vi "testV7-Timer.vi"() -> ()   [LabVIEW 2020]
uses:
  <vilib>/DAQmx/read.llb/DAQmx Read (Analog 2D DBL NChan NSamp).vi
  <vilib>/Analysis/baseanly.llb/Mean (DBL).vi
  <vilib>/DAQmx/miscellaneous.llb/DAQmx Fill In Error Info.vi
  <vilib>/Analysis/NI_AALBase.lvlib
  <resource>/objmgr/daqmx.rc
panel:
  out "index of element":i32
  out "element":dbl
  out "?":timestamp
  out "Channels":refnum<k21>[](array[refnum])
  in  "stop":bool
  out "size(s)":i32
  out "NumDevices":u32
  out "x/y":dbl
  in  "?":T1(tab)
  in  "Sampling Time":u32=5
  in  "Read Time (s)":u32=60
  in  "Channel List":string(combo)="Temperature"
  out "Read Count Daily":string="7/26/2020\n 6:17:48 PM" caption="Timestamp"
  out "Countdown to Read":string="7/26/2020\n 6:17:48 PM" caption="Timestamp"
  out "?":string
  out "?":string
  out "Timestamp":string="7/26/2020\n 6:17:48 PM"
  in  "Play Button 2":bool
  in  "Next Button":bool
  in  "Stop Button 2":bool
  out "Graph Running":bool
  in  "Resolution":u8=10 min=10
  in  "Stop Button":bool
  in  "Play Button":bool
  out "Module 3":bool
  out "Module 2":bool
  out "Module 1":bool
  out "3":bool
  out "2":bool
  out "1":bool
  in  "Running Module":u8=1 min=1 max=3
  in  "Module 3 Task":refnum<k21>="MyTemperatureTask_2"
  out "?":waveform(dbl)(graph)
  in  "Module 3 File Data Location":path=path "E:/KMUTT/Master Degree/labviewjgsee/log/Module3"
  in  "Module 2 File Data Location":path=path "E:/KMUTT/Master Degree/labviewjgsee/log/Module2"
  in  "Module 2 Task":refnum<k21>="MyTemperatureTask_1"
  in  "Module 1 File Data Location":path=path "E:/KMUTT/Master Degree/labviewjgsee/log/Module1"
  in  "Module 1 Task":refnum<k21>="MyTemperatureTask"
  in  "DAQmx Device Name":tag
  out "Table Module 1":string[][](table)
  out "Table Module 2":string[][](table)
  out "Table Module 3":string[][](table)
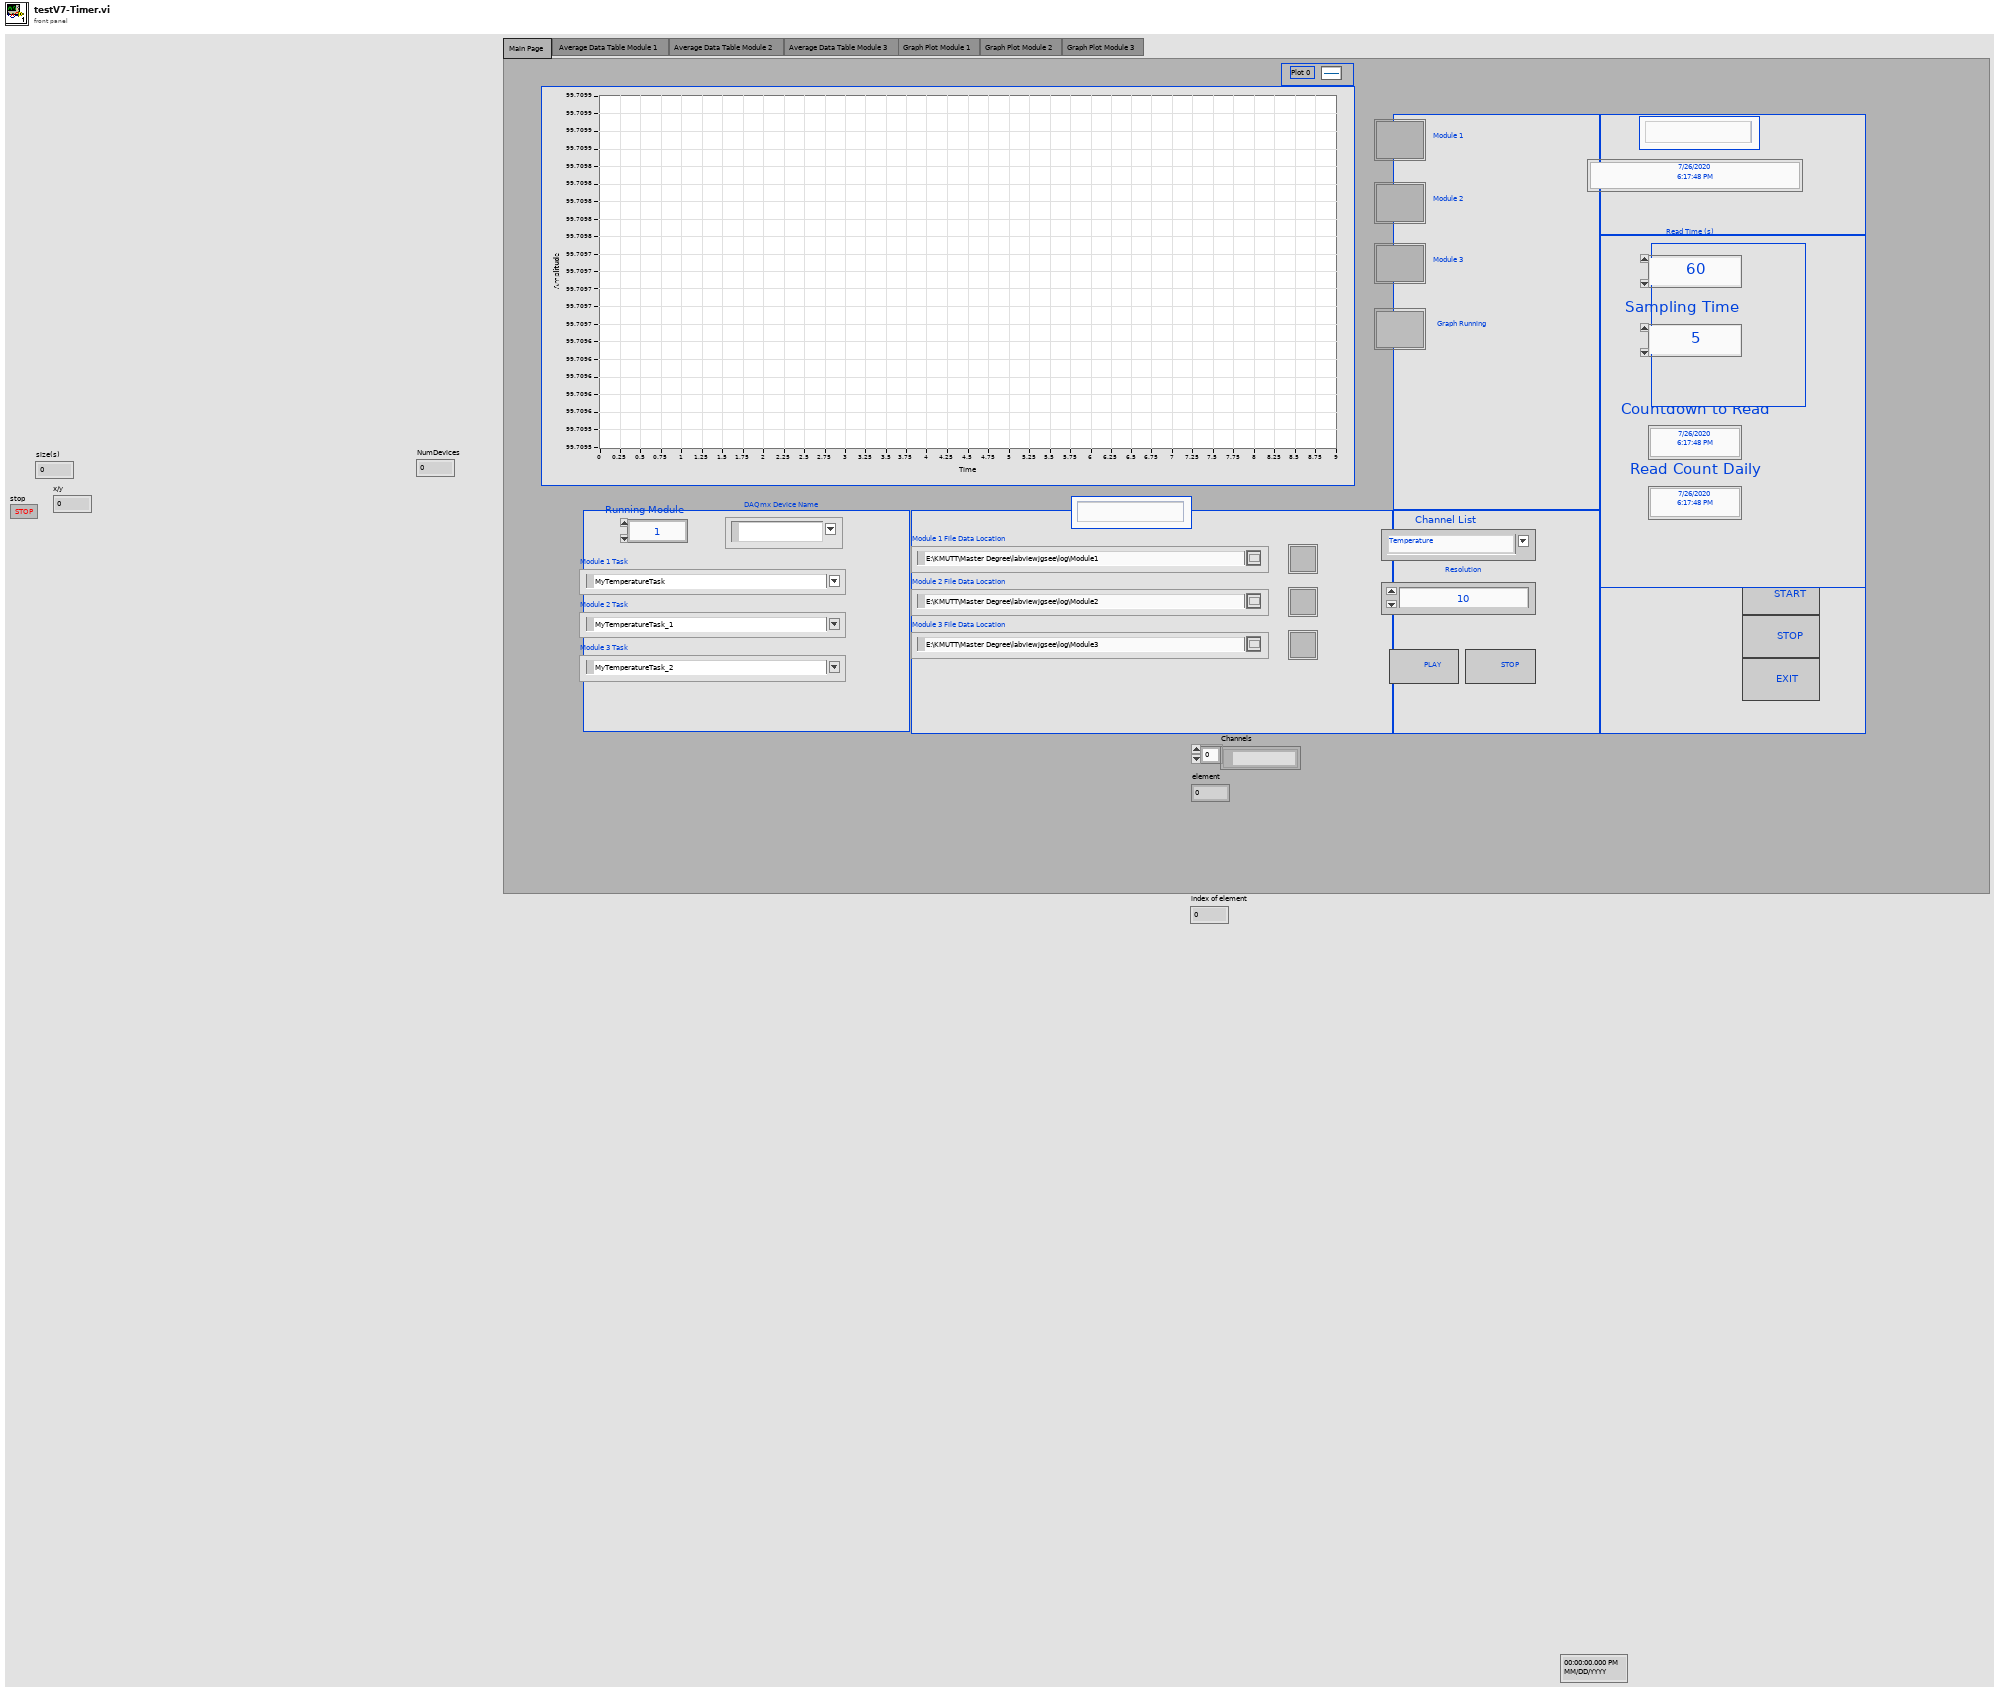
[diagram p1: front panel]
types:
  T1 = enum32{"Main Page ", " Average Data Table Module 1", "Average Data Table Module 2", "Average Data Table Module 3", "Graph Plot Module 1", "Graph Plot Module 2", "Graph Plot Module 3"}
  T2 = enum16{"open", "replace", "create", "open or create", "replace or create", "replace or create with confirmation"}
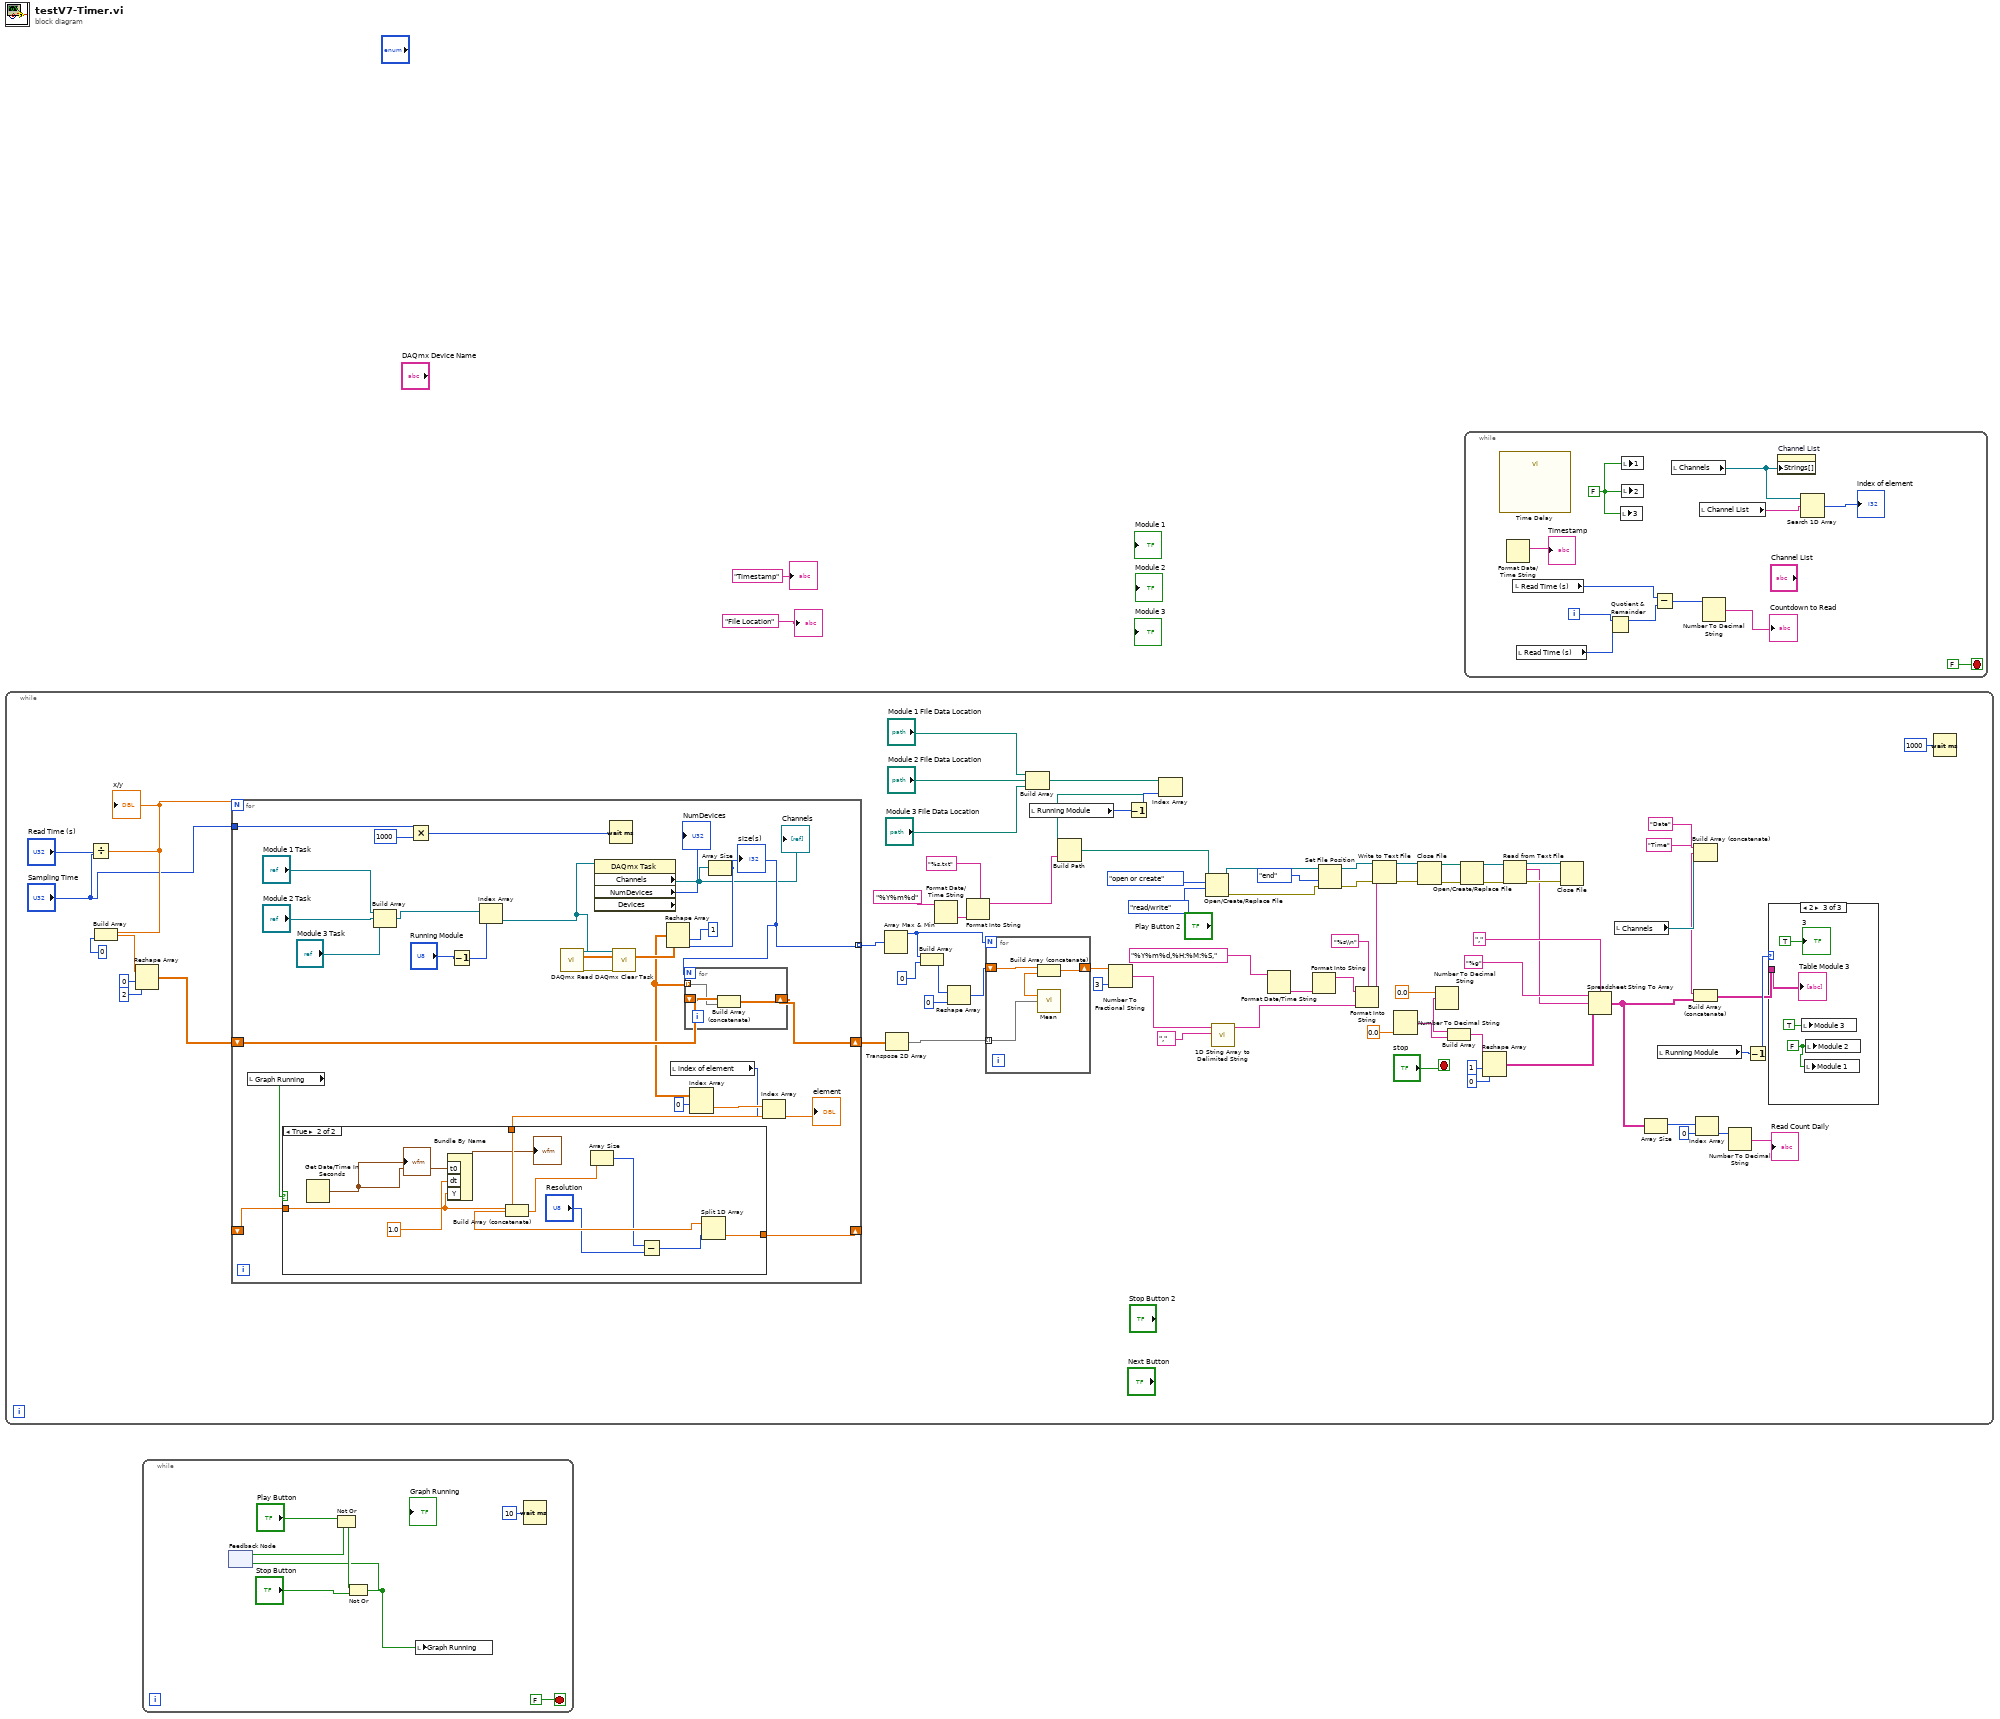
[diagram p0: block diagram]
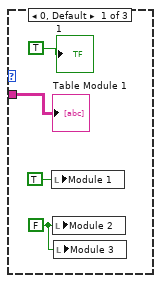
[diagram p2: hidden frame]
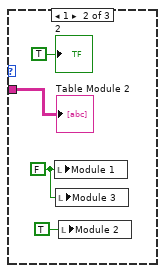
[diagram p3: hidden frame]
diagram:
  n1 = while {
    stop <- "stop" stop-if-true
    n2 = Divide(x="Read Time (s)", y="Sampling Time") -> (x/y=w55:dbl)
    "x/y" <- w55
    n3 = Build Array(w55, 0 ("element")) -> (w59:dbl[])
    n4 = Reshape Array(w59, 0 ("dimension size"), 2 ("dimension size")) -> (w56:dbl[][])
    n5 = for {
      N: w55 -> [_]
      shift-right: [w116] -> w24
      shift-left: w56 -> [w115]
      tunnel: "Sampling Time" -> [w114]
      tunnel: [w112] -> w54 mode=indexing
      shift-right: [w96] -> _
      shift-left: _ -> [w95]
      n6 = local read "Graph Running"() -> (w94:bool)
      n7 = Build Array("Module 1 Task", "Module 2 Task", "Module 3 Task") -> (w107:refnum<k21>[])
      n8 = Multiply(x=w114, y=u32 1000) -> (x*y=w102:u32)
      n9 = Decrement(x="Running Module") -> (x-1=w103:u8)
      n10 = Index Array(array=w107, index=w103) -> (element=w106:refnum<k21>)
      n11 = call-poly <vilib>:"DAQmx Read.vi"("task/channels in"=w106) -> ("task out"=w118:refnum<k21>, "data"=w111:dbl[][], "error out"=w119:errorcluster)  [unwired: 12 in]
      n12 = property class="DAQmx Task" props=["Channels", "NumDevices", "Devices"](reference=w106) -> ("Channels"=w101:refnum<k21>[], "NumDevices"=→"NumDevices":u32)  [unwired: 1 in, 3 out]
      "Channels" <- w101
      n13 = Wait (ms)(milliseconds to wait=w102) -> ()  [unwired: 1 out]
      n14 = call <vilib>:"DAQmx Clear Task.vi"("task in"=w118, "error in"=w119) -> ()  [unwired: 13 in, 1 out]
      n15 = local read "index of element"() -> (w93:i32)
      n16 = Array Size(array=w101) -> (size(s)=w112:i32)
      "size(s)" <- w112
      n17 = Reshape Array(w111, 1 ("dimension size"), w112) -> (w100:dbl[][])
      n18 = for {
        N: w112 -> [_]
        shift-right: [w131] -> w116
        shift-left: w115 -> [w132]
        tunnel: w100 -> [w130] mode=indexing
        n19 = Build Array (concatenate)(w132, w130) -> (w131:dbl[][])
      }
      n20 = Index Array(array=w100, index (row)=0) -> (element=w98:dbl[])  [unwired: 1 in]
      n21 = Index Array(array=w98, index=w93) -> (element=w97:dbl)
      "element" <- w97
      n22 = case shown="True" w94 {
        tunnel: w97 -> [_ w127]
        tunnel: [_ w124] -> w96
        tunnel: w95 -> [_ w123]
        frame False {
        }
        frame True {
          n23 = Get Date/Time In Seconds() -> (seconds since 1Jan1904=w129:timestamp)
          "?" <- w129
          n24 = Bundle By Name("t0"=w129, "dt"=1.0, "Y"=w123) -> (→"?":waveform(dbl))  [unwired: 1 in]
          n25 = Build Array (concatenate)(w123, w127) -> (w125:dbl[])
          n26 = Array Size(array=w125) -> (size(s)=w121:i32)
          n27 = Subtract(x=w121, y="Resolution") -> (x-y=w122:i32)
          n28 = Split 1D Array(array=w125, index=w122) -> (second subarray=w124:dbl[])  [unwired: 1 out]
        }
      }
    }
    n29 = Array Max & Min(array=w54) -> (max value=w51:i32)  [unwired: 3 out]
    n30 = Transpose 2D Array(2D array=w24) -> (transposed array=w53:dbl[][])
    n31 = Build Array(w51, 0 ("element")) -> (w49:i32[])
    n32 = Format Date/Time String(time format string (%c)="%Y%m%d") -> (date/time string=w71:string)  [unwired: 2 in]
    n33 = Reshape Array(w49, 0 ("dimension size")) -> (w48:i32[])
    n34 = Format Into String(format string="%s.txt", w71) -> (resulting string=w69:string)  [unwired: 2 in, 1 out]
    n35 = for {
      N: w51 -> [_]
      tunnel: w53 -> [w136] mode=indexing
      shift-right: [w134] -> w61
      shift-left: w48 -> [w133]
      n36 = call-poly <vilib>:"Mean.vi"("X"=w136) -> ("mean"=w135:dbl)  [unwired: 1 out]
      n37 = Build Array (concatenate)(w133, w135) -> (w134:dbl[])
    }
    n38 = Build Array("Module 1 File Data Location", "Module 2 File Data Location", "Module 3 File Data Location") -> (w17:path[])
    n39 = local read "Running Module"() -> (w18:u8)
    n40 = Number To Fractional String(number=w61, precision (6)=i16 3) -> (F-format string=w62:string[])  [unwired: 2 in]
    n41 = Decrement(x=w18) -> (x-1=w16:u8)
    n42 = Index Array(array=w17, index=w16) -> (element=w15:path)
    n43 = Build Path(base path=w15, name or relative path=w69) -> (appended path=w68:path)
    n44 = Open/Create/Replace File(file path (use dialog)=w68, operation (0:open)=T2."open or create", access (0:read/write)=enum16{"read/write", "read-only", "write-only"}."read/write") -> (refnum out=w46:refnum<file>, error out=w75:errorcluster)  [unwired: 3 in, 1 out]
    n45 = call <vilib>:"1D String Array to Delimited String.vi"("delimiter"="," ("format string"), "string array"=w62) -> ("delimited string"=w67:string)  [unwired: 9 in]
    n46 = Format Date/Time String(time format string (%c)="%Y%m%d,%H:%M:%S,") -> (date/time string=w64:string)  [unwired: 2 in]
    n47 = Format Into String(w64) -> (resulting string=w63:string)  [unwired: 3 in, 1 out]
    n48 = Set File Position(refnum=w46, from (0:start)=enum16{"start", "end", "current"}."end", error in=w75) -> (refnum out=w76:refnum<file>, error out=w74:errorcluster)  [unwired: 1 in]
    n49 = Format Into String(format string="%s\\n", initial string=w63, w67) -> (resulting string=w38:string)  [unwired: 1 in, 1 out]
    n50 = Write to Text File(file (use dialog)=w76, text=w38, error in=w74) -> (refnum out=w45:refnum<file>, error out=w44:errorcluster)  [unwired: 1 in, 1 out]
    n51 = Number To Decimal String(number=0.0 ("element")) -> (decimal integer string=w26:string)  [unwired: 1 in]
    n52 = Close File(refnum=w45, error in=w44) -> (path=w43:path, error out=w42:errorcluster)
    n53 = Number To Decimal String(number=0.0 ("element")) -> (decimal integer string=w28:string)  [unwired: 1 in]
    n54 = Build Array(w28, w26) -> (w30:string[])
    n55 = Open/Create/Replace File(file path (use dialog)=w43, error in=w42) -> (refnum out=w41:refnum<file>, error out=w40:errorcluster)  [unwired: 4 in, 1 out]
    n56 = Reshape Array(w30, 1 ("dimension size"), 0 ("dimension size")) -> (w31:string[][])
    n57 = Read from Text File(file (use dialog)=w41, error in=w40) -> (refnum out=w39:refnum<file>, text=w34:string, error out=w35:errorcluster)  [unwired: 2 in, 1 out]
    n58 = Close File(refnum=w39, error in=w35) -> ()  [unwired: 2 out]
    n59 = Spreadsheet String To Array(delimiter (Tab)=",", format string="%g", spreadsheet string=w34, array type (2D Dbl)=w31) -> (array=w7:string[][])
    n60 = local read "Channels"() -> (w9:refnum<k21>[])
    n61 = Array Size(array=w7) -> (size(s)=w6:i32[])
    n62 = local read "Running Module"() -> (w14:u8)
    n63 = Build Array (concatenate)("Date", "Time", w9) -> (w8:string[])
    n64 = Build Array (concatenate)(w8, w7) -> (w12:string[][])
    n65 = Index Array(array=w6, index=0) -> (element=w4:i32)
    n66 = Number To Decimal String(number=w4) -> (decimal integer string=→"Read Count Daily":string)  [unwired: 1 in]
    n67 = Decrement(x=w14) -> (x-1=w13:u8)
    n68 = case shown="2" w13 {
      tunnel: w12 -> [w84 w88 w92]
      frame 0, Default {
        w81 = FALSE ("Module 2")
        n69 = local write "Module 1"(TRUE ("Module 1")) -> ()
        n70 = local write "Module 2"(w81) -> ()
        n71 = local write "Module 3"(w81) -> ()
        "Table Module 1" <- w84
        "1" <- TRUE ("1")
      }
      frame 1 {
        w85 = FALSE ("Module 1")
        n72 = local write "Module 1"(w85) -> ()
        n73 = local write "Module 3"(w85) -> ()
        n74 = local write "Module 2"(TRUE ("Module 2")) -> ()
        "Table Module 2" <- w88
        "2" <- TRUE ("2")
      }
      frame 2 {
        w89 = FALSE ("Module 2")
        n75 = local write "Module 3"(TRUE ("Module 3")) -> ()
        n76 = local write "Module 1"(w89) -> ()
        n77 = local write "Module 2"(w89) -> ()
        "Table Module 3" <- w92
        "3" <- TRUE ("3")
      }
    }
    n78 = Wait (ms)(milliseconds to wait=u32 1000) -> ()  [unwired: 1 out]
  }
  n79 = while {
    stop <- FALSE stop-if-true
    n80 = feedback #1() -> (w138:bool)  [unwired: 1 in]
    n81 = Not Or(1:w138, 2:"Play Button") -> (0:w139:bool)
    n82 = Not Or(1:"Stop Button", 2:w139) -> (0:w137:bool)
    n83 = feedback-in #1(w137) -> ()
    n84 = local write "Graph Running"(w137) -> ()
    n85 = Wait (ms)(milliseconds to wait=u32 10) -> ()  [unwired: 1 out]
  }
  n86 = while {
    i -> [w152]
    stop <- FALSE stop-if-true
    w155 = FALSE ("1")
    n87 = call "Time Delay"() -> ()  [unwired: 11 in, 1 out]
    n88 = Format Date/Time String() -> (date/time string=→"Timestamp":string)  [unwired: 3 in]
    n89 = local read "Read Time (s)"() -> (w149:u32)
    n90 = local read "Read Time (s)"() -> (w151:u32)
    n91 = Quotient & Remainder(x=w152, y=w151) -> (x-y*floor(x/y)=w150:u32)  [unwired: 1 out]
    n92 = local write "3"(w155) -> ()
    n93 = local write "1"(w155) -> ()
    n94 = local write "2"(w155) -> ()
    n95 = Subtract(x=w149, y=w150) -> (x-y=w148:u32)
    n96 = local read "Channels"() -> (w146:refnum<k21>[])
    n97 = local read "Channel List"() -> (w145:string)
    n98 = Number To Decimal String(number=w148) -> (decimal integer string=→"Countdown to Read":string)  [unwired: 1 in]
    n99 = property on="Channel List" class="CmbBox"("Strings[]"=w146) -> ()  [unwired: 2 in, 2 out]
    n100 = Search 1D Array(1D array=w146, element=w145) -> (index of element=→"index of element":i32)  [unwired: 1 in]
  }
  "?" <- "File Location" ("String")
  "?" <- "Timestamp"
